vi "6-3 Read.vi"() -> ()   [LabVIEW 2017]
panel:
  out "Waveform Chart":dbl(graph)
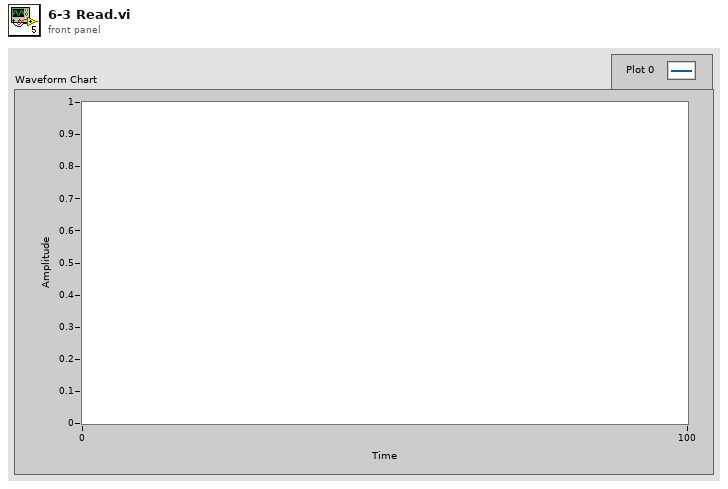
[diagram p1: front panel]
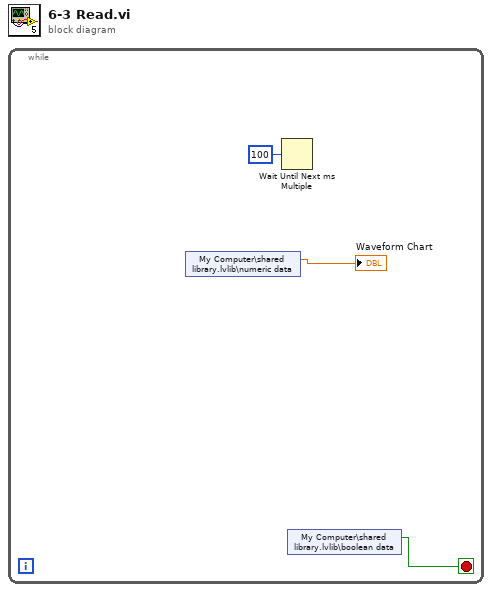
[diagram p0: block diagram]
diagram:
  n1 = while {
    stop <- w3 stop-if-true
    n2 = shared-variable "My Computer\\shared library.lvlib\\numeric data"() -> (→"Waveform Chart":dbl)  [unwired: 1 in, 1 out]
    n3 = Wait Until Next ms Multiple(millisecond multiple=u32 100) -> ()  [unwired: 1 out]
    n4 = shared-variable "My Computer\\shared library.lvlib\\boolean data"() -> (w3:bool)  [unwired: 1 in, 1 out]
  }
